vi "ConvertStatusRegistersToAxisStatusArray.vi"(0 "Array of StatusRegister":T4[](array[typedef]), 5 "error in":errorcluster) -> (14 "Array of AxisStatus":T1[](array[typedef]) {"Drive State Machine" items=["Ready to Switch On"=0, "Fault"=1, "Operation Enabled"=2, "Fault Reaction Active"=3, "Quick Stop Active"=6]}, 19 "error out":errorcluster)   [LabVIEW 2026]
uses:
  GeneralCommands/Status.ctl
  GeneralCommands/AxisStatus.ctl
  SpecialCommand/DriveStateMachine.ctl
  SpecialCommand/ModeOfOperation.ctl
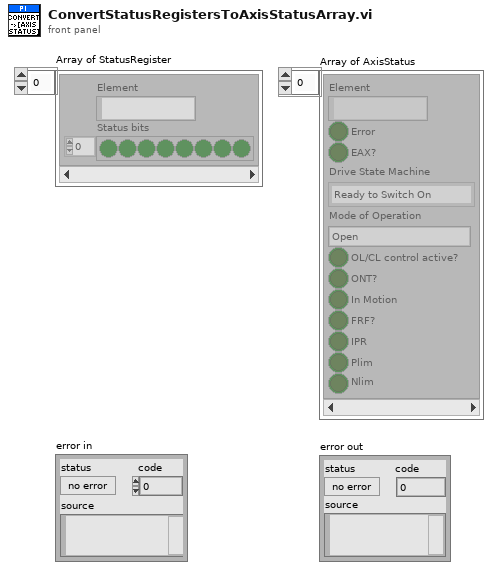
[diagram p1: front panel]
types:
  T1 = typedef "AxisStatus.ctl" = cluster{"Element":string, "Error":bool, "EAX?":bool, "Drive State Machine":T2, "Mode of Operation":T3, "OL/CL control active?":bool, "ONT?":bool, "In Motion":bool, "FRF?":bool, "IPR":bool, "Plim":bool, "Nlim":bool}
  T2 = typedef "DriveStateMachine.ctl" = u16
  T3 = typedef "ModeOfOperation.ctl" = enum16{"Open", "Open-Loop Position", "Closed-Loop Position", "Open-Loop Velocity", "Closed-Loop Velocity", "Open-Loop Force", "Closed-Loop Force", "Step Operation"}
  T4 = typedef "Status.ctl" = cluster{"Element":string, "Status bits":bool[]}
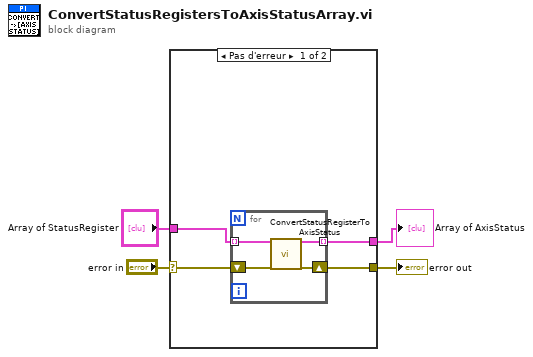
[diagram p0: block diagram]
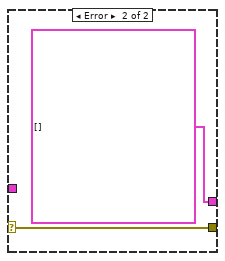
[diagram p2: hidden frame]
diagram:
  n1 = case shown="Pas d'erreur" "error in" {
    selector: "error in" -> [w8 w14]
    tunnel: [w7 w14] -> w3
    tunnel: "Array of StatusRegister" -> [w6 _]
    tunnel: [w5 T1[] []] -> w1
    frame No Error {
      n2 = for {
        shift-right: [w12] -> w7
        shift-left: w8 -> [w11]
        tunnel: w6 -> [w10] mode=indexing
        tunnel: [w9] -> w5 mode=indexing
        n3 = call "ConvertStatusRegisterToAxisStatus.vi"("Status"=w10, "error in"=w11) -> ("AxisStatus"=w9:T1, "error out"=w12:errorcluster)  [unwired: 16 in]
      }
    }
    frame Error {
    }
  }
  "error out" <- w3
  "Array of AxisStatus" <- w1
